vi "Get Type.vi"(8 "error in (no error)":errorcluster, 11 "Electronic Parts in":refnum<class "Electronic Parts.lvclass">) -> (0 "error out":errorcluster, 2 "Item Type":T1, 3 "Electronic Parts out":refnum<class "Electronic Parts.lvclass">)   [LabVIEW 2020, in "Electronic Parts.lvclass"]
uses:
  Electronic Parts.lvclass
  Item/Item Type.ctl
  Item/Item.lvclass
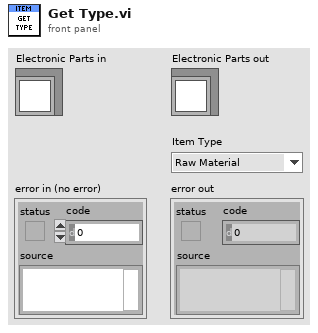
[diagram p1: front panel]
types:
  T1 = typedef "Item.lvclass/Item Type.ctl" = enum16{"Raw Material", "Component", "Module", "Product"}
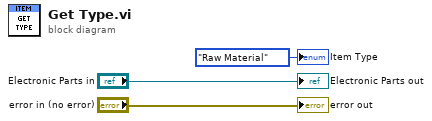
[diagram p0: block diagram]
diagram:
  "error out" <- "error in (no error)"
  "Electronic Parts out" <- "Electronic Parts in"
  "Item Type" <- Item_Type."Raw Material" ("Item Type")
